vi "stitchingModeSimple.vi"(7 "Data In":dbl[][](array[numeric]), 8 "Pixel overlap":i32=100, 9 "X Pixels:":i32=1024, 10 "Iterations":i32) -> (2 "Data Out":dbl[][](array[numeric]))   [LabVIEW 2023, in "horiba.lvlib" / "CCD.lvclass"]
uses:
  CCD.lvclass
  CCD.lvclass/CCD.ctl
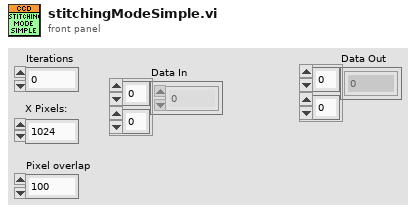
[diagram p1: front panel]
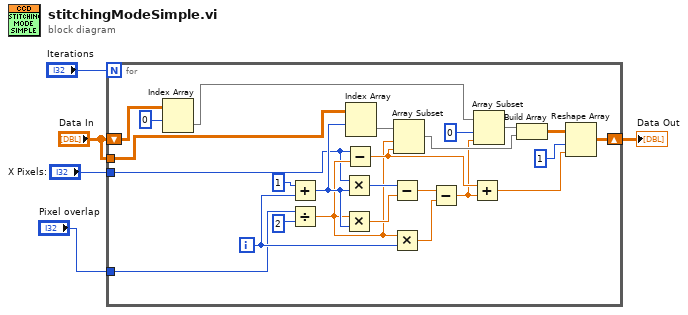
[diagram p0: block diagram]
diagram:
  n1 = for {
    N: "Iterations" -> [_]
    shift-right: [w17] -> w5
    shift-left: "Data In" -> [w30]
    tunnel: "Data In" -> [w28]
    tunnel: "Pixel overlap" -> [w7]
    tunnel: "X Pixels:" -> [w6]
    i -> [w11]
    n2 = Index Array(array=w30, index (row)=0) -> (element=w27:dbl[])  [unwired: 1 in]
    n3 = Add(x=1, y=w11) -> (x+y=w13:i32)
    n4 = Divide(x=w7, y=2) -> (x/y=w8:dbl)
    n5 = Multiply(x=w6, y=w13) -> (x*y=w16:i32)
    n6 = Multiply(x=w8, y=w13) -> (x*y=w15:dbl)
    n7 = Subtract(x=w6, y=w8) -> (x-y=w14:dbl)
    n8 = Index Array(array=w28, index (row)=w13) -> (element=w24:dbl[])  [unwired: 1 in]
    n9 = Subtract(x=w16, y=w15) -> (x-y=w12:dbl)
    n10 = Multiply(x=w8, y=w11) -> (x*y=w10:dbl)
    n11 = Array Subset(array=w24, index=w8, length=w14) -> (w21:dbl[])
    n12 = Subtract(x=w12, y=w10) -> (x-y=w9:dbl)
    n13 = Add(x=w14, y=w9) -> (x+y=w18:dbl)
    n14 = Array Subset(array=w27, index=0, length=w9) -> (w22:dbl[])
    n15 = Build Array(w22, w21) -> (w20:dbl[][])
    n16 = Reshape Array(w20, 1 ("dimension size"), w18) -> (w17:dbl[][])
  }
  "Data Out" <- w5
